vi "Stream Pause.vi"(8 "error in":errorcluster, 9 "Pause?":bool, 11 "UART port in":T1) -> (0 "error out":errorcluster, 3 "UART port out":T1)   [LabVIEW 2015]
doc: "Pause or resume an active sensor stream.\n\nThis VI writes to, but does not read from, the serial port."
uses:
  Advanced/UART/iRobot UART Port Type.ctl
  Advanced/Command/OpCode.ctl
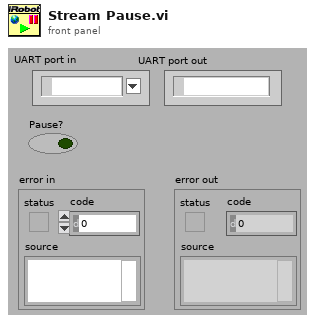
[diagram p1: front panel]
types:
  T1 = typedef "iRobot UART Port Type.ctl" = refnum<visa-resource-name>
  T2 = typedef "OpCode.ctl" = u8
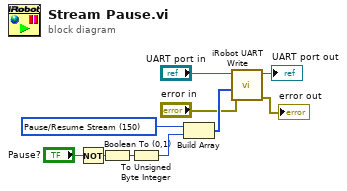
[diagram p0: block diagram]
diagram:
  w9 = T2 150 items=["Start"=128, "Baud"=129, "Control"=130, "Safe"=131, "Full"=132, "Demo"=136, "Demo - Cover"=135, "Demo - Cover and Dock"=143, "Demo - Spot"=134, "Drive"=137, "Drive Direct"=145, "LEDs"=139, "Digital Outputs"=147, "PWM Low Side Drivers"=144, "Low Side Drivers"=138, "Send IR"=151, "Song"=140, "Play Song"=141, "Sensors"=142, "Query List"=149, "Stream"=148, "Pause/Resume Stream"=150, "Script"=152, "Play Script"=153, "Show Script"=154, "Wait Time"=155, "Wait Distance"=156, "Wait Angle"=157, "Wait Event"=158] ("OpCode")
  n1 = Not(x="Pause?") -> (.not. x?=w2:bool)
  n2 = Boolean To (0,1)(Boolean=w2) -> (0, 1=w8:i16)
  n3 = To Unsigned Byte Integer(number=w8) -> (unsigned 8bit integer=w1:u8)
  n4 = Build Array(w9, w1) -> (w7:T2[])
  n5 = call "iRobot UART Write.vi"("error in"="error in", "data"=w7, "UART port in"="UART port in") -> ("error out"=→"error out":errorcluster, "UART port out"=→"UART port out":T1)  [unwired: 1 in, 6 out]
